vi "testAbortVI.vi"(8 "error in (no error)":errorcluster, 11 "TestCase in":refnum<class "Abort Application Unit Test.lvclass">) -> (0 "error out":errorcluster, 3 "TestCase out":refnum<class "Abort Application Unit Test.lvclass">)   [LabVIEW 2016, in "Assert API Components.lvlib" / "Log Assert Core.lvlib" / "Abort Application Unit Test.lvclass"]
uses:
  Abort Application Unit Test.lvclass
  Core/Assert API Components/Message Data.ctl
  Core/Assert API Components/Failure Actions.ctl
  Core/Assert API Components/VI References.ctl
  <vilib>/addons/_JKI Toolkits/VI Tester/TestCase.llb/TestCase.lvclass
  Core/Assert API Components/Assert API Components.lvlib
  Call Abort VI.vi
  C:/Program Files (x86)/National Instruments/LabVIEW 2016/vi.lib/addons/_JKI Toolkits/VI Tester/TestCase.llb/TestCase.lvclass
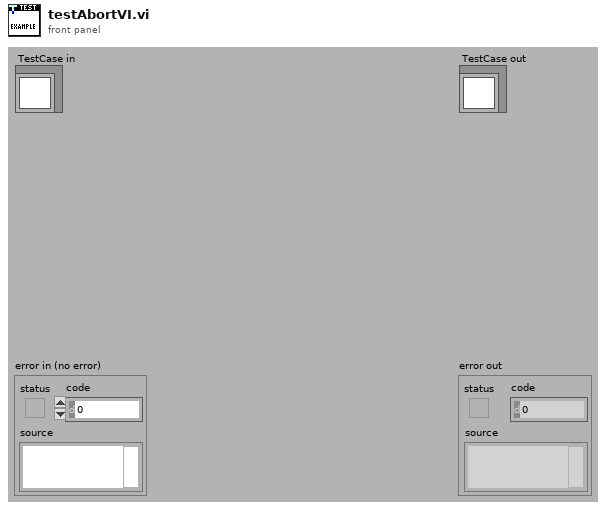
[diagram p1: front panel]
types:
  T1 = enum32{"Invalid", "Standard", "Closed", "Hidden", "Minimized", "Maximized"}
  T2 = typedef "Assert API Components.lvlib/Message Data.ctl" = cluster{"Data Value":variant, "Last Update":timestamp, "Comment":string, "Evaluation String":string, "Status":bool, "Assert Name":string, "Failure Action":T3, "Assert VI Name":string, "Calling VI Name":string, "Assert VI UID":i32, "Top Level VI Name":string, "VI References":T4, "Assert Build Timestamp":timestamp, "Assert Builder User Name":string, "Data Type":string, "IP Address":string}
  T3 = typedef "Assert API Components.lvlib/Failure Actions.ctl" = enum16{"None", "Log To File", "Pause Execution", "Abort Execution"}
  T4 = typedef "Assert API Components.lvlib/VI References.ctl" = cluster{"Calling VI Ref":refnum<vi>, "Assert VI Ref":refnum<vi>}
  T5 = enum32{"Bad", "Idle", "Run top level", "Running"}
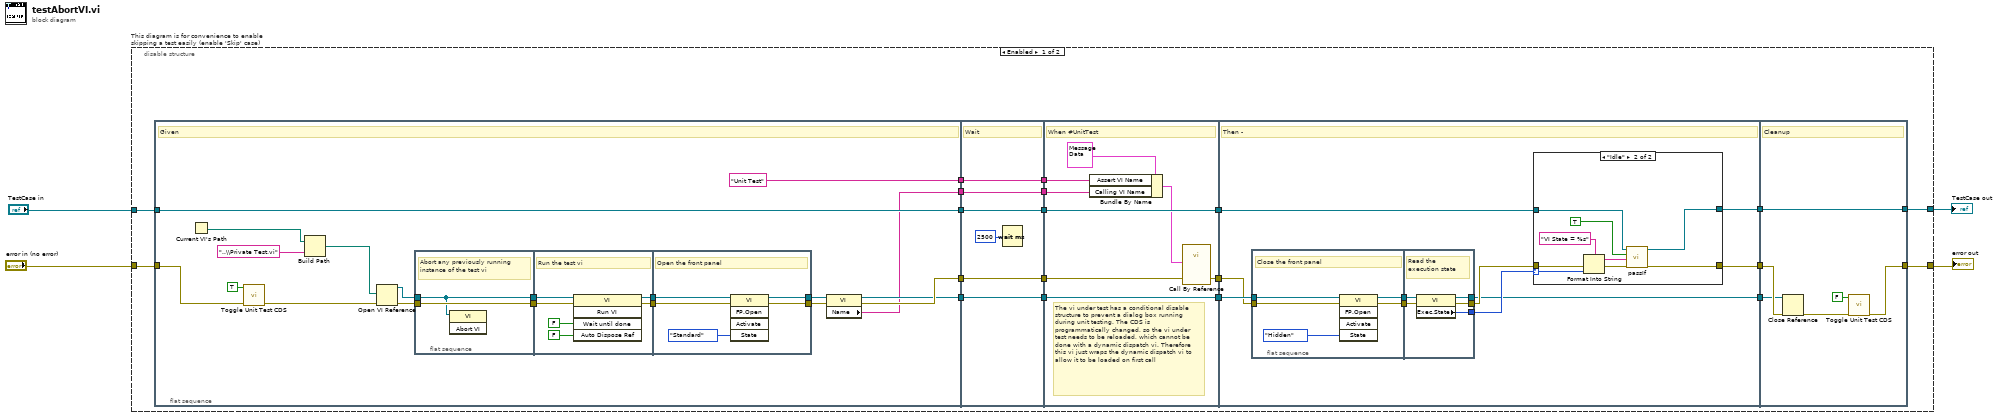
[diagram p0: block diagram]
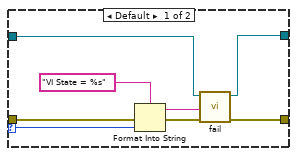
[diagram p2: hidden frame]
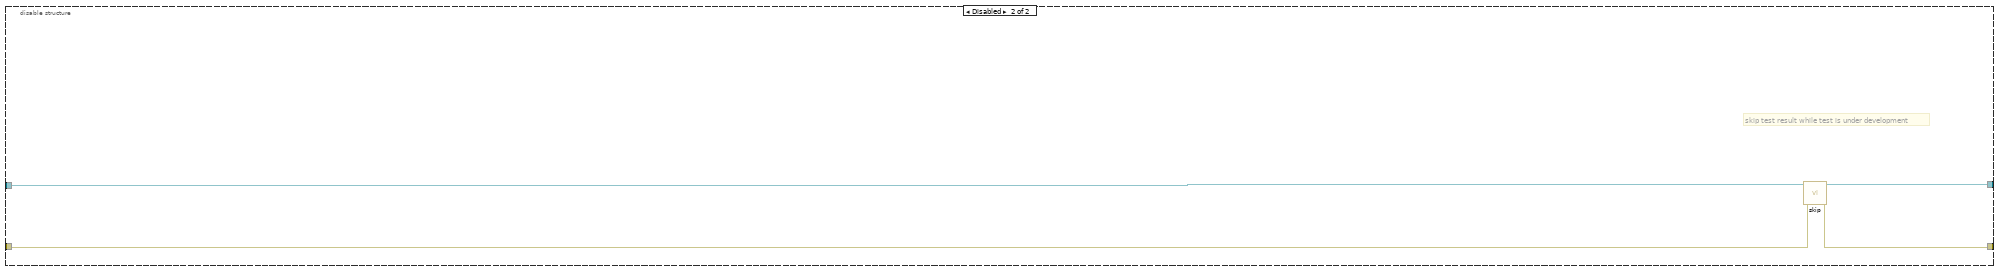
[diagram p3: hidden frame]
diagram:
  n1 = disable-structure "This diagram is for convenience to enable skipping a test easily (enable 'Skip' case)" shown="Enabled" {
    disable-tunnel: "TestCase in" -> [w23 w117]
    disable-tunnel: [w20 w115] -> w1
    disable-tunnel: [w22 w116] -> w3
    disable-tunnel: "error in (no error)" -> [w18 w114]
    frame Enabled {
      n2 = flat-sequence {
        tunnel: w23 -> [w43]
        tunnel: [w43] -> w17
        tunnel: w18 -> [w27]
        tunnel: [w31] -> w15
        tunnel: [w28] -> w12
        tunnel: ["Unit Test" ("Assert VI Name")] -> w10
        tunnel: [w29] -> w6
        tunnel: w17 -> [w62]
        tunnel: [w62] -> w16
        tunnel: w15 -> [w60]
        tunnel: [w60] -> w14
        tunnel: [w59] -> w13
        tunnel: w12 -> [w59]
        tunnel: [w58] -> w11
        tunnel: w10 -> [w58]
        tunnel: [w57] -> w7
        tunnel: w6 -> [w57]
        tunnel: [w70] -> w24
        tunnel: w16 -> [w70]
        tunnel: w14 -> [w69]
        tunnel: w13 -> [w64]
        tunnel: w11 -> [w68]
        tunnel: [w66] -> w9
        tunnel: [w65] -> w8
        tunnel: w7 -> [w65]
        tunnel: w24 -> [w75]
        tunnel: [w80] -> w21
        tunnel: [w79] -> w19
        tunnel: w9 -> [w77]
        tunnel: w8 -> [w78]
        tunnel: [w73] -> w5
        tunnel: [w109] -> w22
        tunnel: w21 -> [w112]
        tunnel: [w113] -> w20
        tunnel: w19 -> [w113]
        tunnel: w5 -> [w111]
        frame #0 {
          # "Given"
          n3 = Current VI's Path() -> (path=w39:path)
          n4 = call "Toggle Unit Test CDS.vi"("error in (no error)"=w27, "Requested State"=TRUE) -> ("error out"=w26:errorcluster)  [unwired: 9 in]
          n5 = Build Path(base path=w39, name or relative path="..\\Private Test.vi") -> (appended path=w38:path)
          n6 = Open VI Reference(vi path=w38, error in (no error)=w26) -> (vi reference=w36:refnum<vi>, error out=w35:errorcluster)  [unwired: 4 in]
          n7 = flat-sequence {
            tunnel: [w45] -> w37
            tunnel: w36 -> [w44]
            tunnel: w35 -> [w45]
            tunnel: [w44] -> w34
            tunnel: w37 -> [w47]
            tunnel: w34 -> [w46]
            tunnel: [w49] -> w33
            tunnel: [w48] -> w32
            tunnel: [w53] -> w30
            tunnel: [w55] -> w42
            tunnel: w33 -> [w56]
            tunnel: w32 -> [w54]
            frame #0 {
              # "Abort any previously running instance of the test vi"
              n8 = invoke class="VI" method="Abort VI"(reference=w44) -> ()  [unwired: 2 in, 3 out]
            }
            frame #1 {
              # "Run the test vi"
              n9 = invoke class="VI" method="Run VI"(reference=w46, error in=w47, "Wait until done"=FALSE ("Wait Until Done"), "Auto Dispose Ref"=FALSE ("Auto Dispose Reference")) -> (reference out=w48:refnum<vi>, error out=w49:errorcluster)  [unwired: 1 in, 3 out]
            }
            frame #2 {
              # "Open the front panel"
              n10 = invoke class="VI" method="FP.Open"(reference=w54, error in=w56, "State"=T1."Standard") -> (reference out=w53:refnum<vi>, error out=w55:errorcluster)  [unwired: 2 in, 3 out]
            }
          }
          n11 = property class="VI"(reference=w30, error in=w42) -> (reference out=w29:refnum<vi>, error out=w31:errorcluster, "Name"=w28:string)
        }
        frame #1 {
          # "Wait"
          n12 = Wait (ms)(milliseconds to wait=u32 2500) -> ()  [unwired: 1 out]
        }
        frame #2 {
          # "The vi under test has a conditional disable structure to prevent a dialog box running during unit testing. The CDS is programmatically changed, so the vi under test needs to be reloaded, which cannot be done with a dynamic dispatch vi. Therefore this vi just wraps the dynamic dispatch vi to allow it to be loaded on first call"
          # "When #UnitTest"
          n13 = Bundle By Name(cluster=T2 {"Data Value"=variant, "Last Update"=timestamp(0 s since 1904-01-01), "Comment"="", "Evaluation String"="", "Status"=FALSE, "Assert Name"="", "Failure Action"=enum."None", "Assert VI Name"="", "Calling VI Name"="", "Assert VI UID"=0, "Top Level VI Name"="", "VI References"={"Calling VI Ref"=refnum, "Assert VI Ref"=refnum}, "Assert Build Timestamp"=timestamp(0 s since 1904-01-01), "Assert Builder User Name"="", "Data Type"="", "IP Address"=""} ("Assert Message"), "Assert VI Name"=w68, "Calling VI Name"=w64) -> (w67:T2)
          n14 = call-by-ref "?"("error in (no error)"=w69, "Assert Message"=w67) -> ("error out"=w66:errorcluster)  [unwired: 11 in, 2 out]
        }
        frame #3 {
          # "Then -"
          n15 = flat-sequence {
            tunnel: w77 -> [w85]
            tunnel: w78 -> [w83]
            tunnel: [w82] -> w72
            tunnel: [w84] -> w71
            tunnel: [w88] -> w76
            tunnel: [w87] -> w74
            tunnel: [w86] -> w73
            tunnel: w72 -> [w90]
            tunnel: w71 -> [w89]
            frame #0 {
              # "Close the front panel"
              n16 = invoke class="VI" method="FP.Open"(reference=w83, error in=w85, "State"=T1."Hidden") -> (reference out=w82:refnum<vi>, error out=w84:errorcluster)  [unwired: 2 in, 3 out]
            }
            frame #1 {
              # "Read the execution state"
              n17 = property class="VI"(reference=w90, error in=w89) -> (reference out=w86:refnum<vi>, error out=w87:errorcluster, "Exec.State"=w88:T5)
            }
          }
          n18 = case shown="\"Idle\"" w76 {
            selector: w76 -> [w96 w101]
            tunnel: [w92 w107] -> w79
            tunnel: [w91 w106] -> w80
            tunnel: w74 -> [w98 w105]
            tunnel: w75 -> [w93 w104]
            frame Default {
              n19 = Format Into String(format string="VI State = %s", error in=w98, w96) -> (resulting string=w94:string, error out=w97:errorcluster)  [unwired: 1 in]
              n20 = call-dynamic "fail.vi"("error in (no error)"=w97, "message (\"\")"=w94, "TestCase in"=w93) -> ("error out"=w91:errorcluster, "TestCase out"=w92:refnum<class "Abort Application Unit Test.lvclass">)  [unwired: 7 in]
            }
            frame "Idle" {
              n21 = Format Into String(format string="VI State = %s", error in=w105, w101) -> (resulting string=w100:string, error out=w102:errorcluster)  [unwired: 1 in]
              n22 = call-dynamic "passIf.vi"("error in (no error)"=w102, "message (\"\")"=w100, "pass"=TRUE, "TestCase in"=w104) -> ("error out"=w106:errorcluster, "TestCase out"=w107:refnum<class "Abort Application Unit Test.lvclass">)  [unwired: 6 in]
            }
          }
        }
        frame #4 {
          # "Cleanup"
          n23 = Close Reference(reference=w111, error in (no error)=w112) -> (error out=w110:errorcluster)
          n24 = call "Toggle Unit Test CDS.vi"("error in (no error)"=w110, "Requested State"=FALSE) -> ("error out"=w109:errorcluster)  [unwired: 9 in]
        }
      }
    }
    frame Disabled {
      # "skip test result while test is under development"
      n25 = call <vilib>:"skip.vi"("error in (no error)"=w114, "TestCase in"=w117) -> ("error out"=w116:errorcluster, "TestCase out"=w115:refnum<class "Abort Application Unit Test.lvclass">)  [unwired: 8 in]
    }
  }
  "error out" <- w3
  "TestCase out" <- w1
